vi "PDU GUI Configure.vi"(8 "error in (no error)":errorcluster, 11 "Orion PDU in":refnum<class "Orion PDU.lvclass">) -> (0 "error out":errorcluster, 3 "Orion PDU out":refnum<class "Orion PDU.lvclass">)   [LabVIEW 2022 SP3, in "Orion PDU.lvclass"]
uses:
  Orion PDU.lvclass
  Orion PDU.lvclass/Orion PDU.ctl
  Power Distribution.lvclass
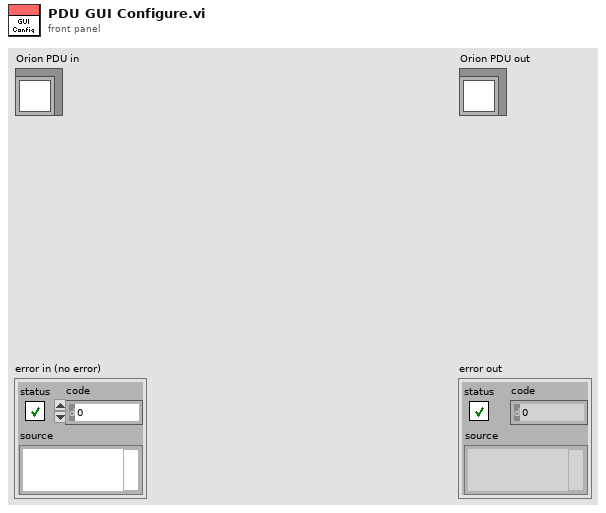
[diagram p1: front panel]
types:
  T1 = typedef "Orion PDU.lvclass/typedef Orion PDU Settings.ctl" = cluster{"URL":string, "Username":string, "Password":string}
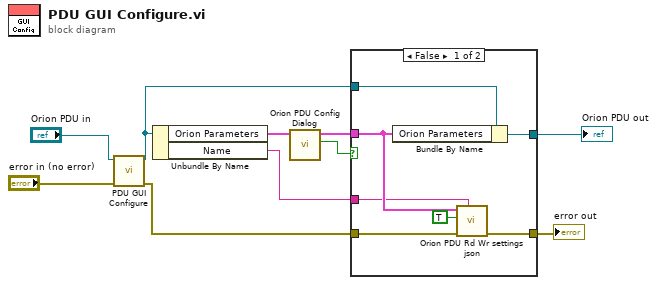
[diagram p0: block diagram]
diagram:
  n1 = call-parent "PDU GUI Configure.vi"("error in (no error)"="error in (no error)", "Power Distribution in"="Orion PDU in") -> ("error out"=w4:errorcluster, "Power Distribution out"=w1:refnum<class "Orion PDU.lvclass">)  [unwired: 8 in]
  n2 = Unbundle By Name(w1) -> ("Orion Parameters"=w9:T1, "Name"=w5:string)
  n3 = call "Orion PDU Config Dialog.vi"("Orion Parameters"=w9) -> ("Cancelled?"=w8:bool, "Orion Parameters out"=w7:T1)  [unwired: 9 in]
  n4 = case shown="False" w8 {
    tunnel: w1 -> [w17 w19]
    tunnel: w7 -> [w15 _]
    tunnel: [w16 w19] -> w6
    tunnel: w5 -> [w14 _]
    tunnel: w4 -> [w12 w18]
    tunnel: [w11 w18] -> w3
    frame False {
      n5 = Bundle By Name(cluster=w17, "Orion Parameters"=w15) -> (w16:refnum<class "Orion PDU.lvclass">)
      n6 = call "Orion PDU Rd Wr settings json.vi"("Name"=w14, "error in (no error)"=w12, "Write? (F:Read)"=TRUE, "Orion Parameters"=w15) -> ("error out"=w11:errorcluster)  [unwired: 6 in, 1 out]
    }
    frame True {
    }
  }
  "error out" <- w3
  "Orion PDU out" <- w6
